vi "Error Strings Global Internal.vi"() -> ()   [LabVIEW 2020]
panel:
  out "5068":string="Couldn't start the measurement service. Please ensure if MeasurementLink is installed or corrupted."
  out "5065":string="Attempted to use session reservation that has been unreserved."
  out "5064":string="No connections found for pins or pin groups '%s' with instrument type id '%s'."
  out "5063":string="No connections found for instrument type id '%s'."
  out "5062":string="Expected a single connection. Found %d connections."
  out "5061":string="Found zero sessions to create."
  out "5060":string="The IInstrument provided an empty Instrument Type ID. Creating sessions requires a valid Instrument Type ID."
  out "5059":string="Attempted to create session for \"%s\" but session already exists."
  out "5058":string="Expected to create exactly 1 session but found %d sessions."
  out "5057":string="Invalid measurement metadata. The following parameter names in `Get Type Specializations.vi` do not match any controls in  `Measurement Configuration.ctl`:"
  out "5056":string="Timed out waiting for discovery service to start."
  out "5055":string="Failed to read the discovery service key file."
  out "5054":string="Failed to get the discovery service key file size."
  out "5053":string="Failed to read the discovery service key file.\nEnsure that the discovery service is running."
  out "5052":string="The %s driver is not installed."
  out "5051":string="LabVIEW cluster contains a type '%s' which is not supported in gRPC."
  out "5050":string="The data type of the following controls are not supported by the Measurement Service.\n\n%s"
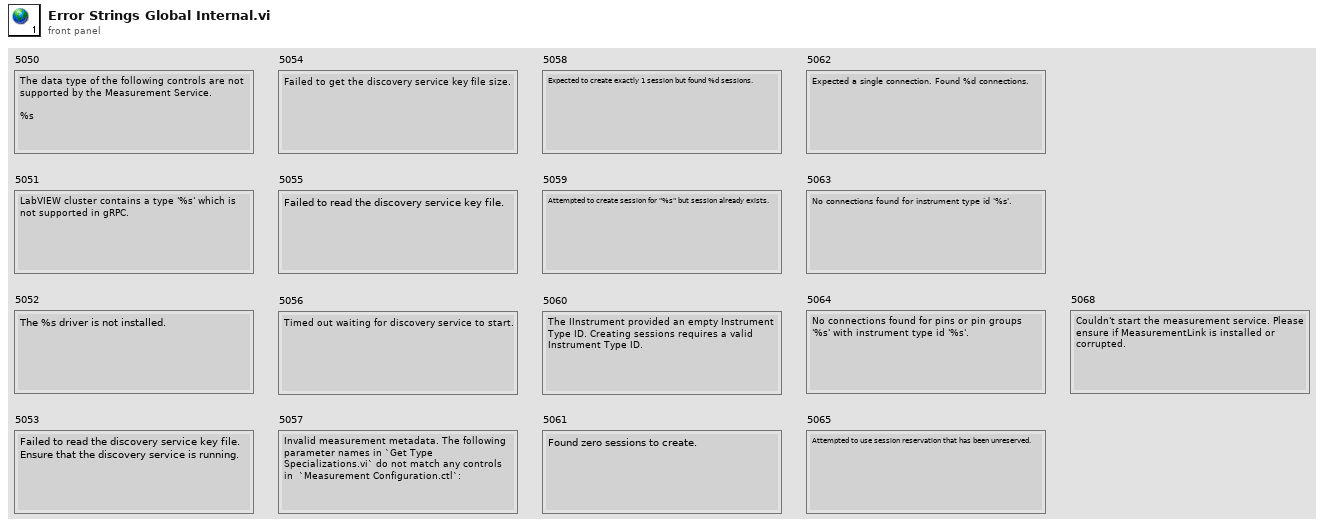
[diagram p1: front panel]
diagram:
